vi "CreateVIPictures.vi"(8 "error in (no error)":errorcluster, 9 "Capture Target":T3=enum."Front Panel", 10 "VI Screenshots":T1, 11 "Picture Save Location":path) -> (0 "error out":errorcluster, 2 "Screenshot Files":path[](array[path]))   [LabVIEW 2017]
doc: "Captures .png imgaes of the VI given the path and the picture configuration."
uses:
  Utilities/FilePaths.ctl
  Screenshot Type.ctl
  ScreenshotInfo.ctl
  VIScreenshots.ctl
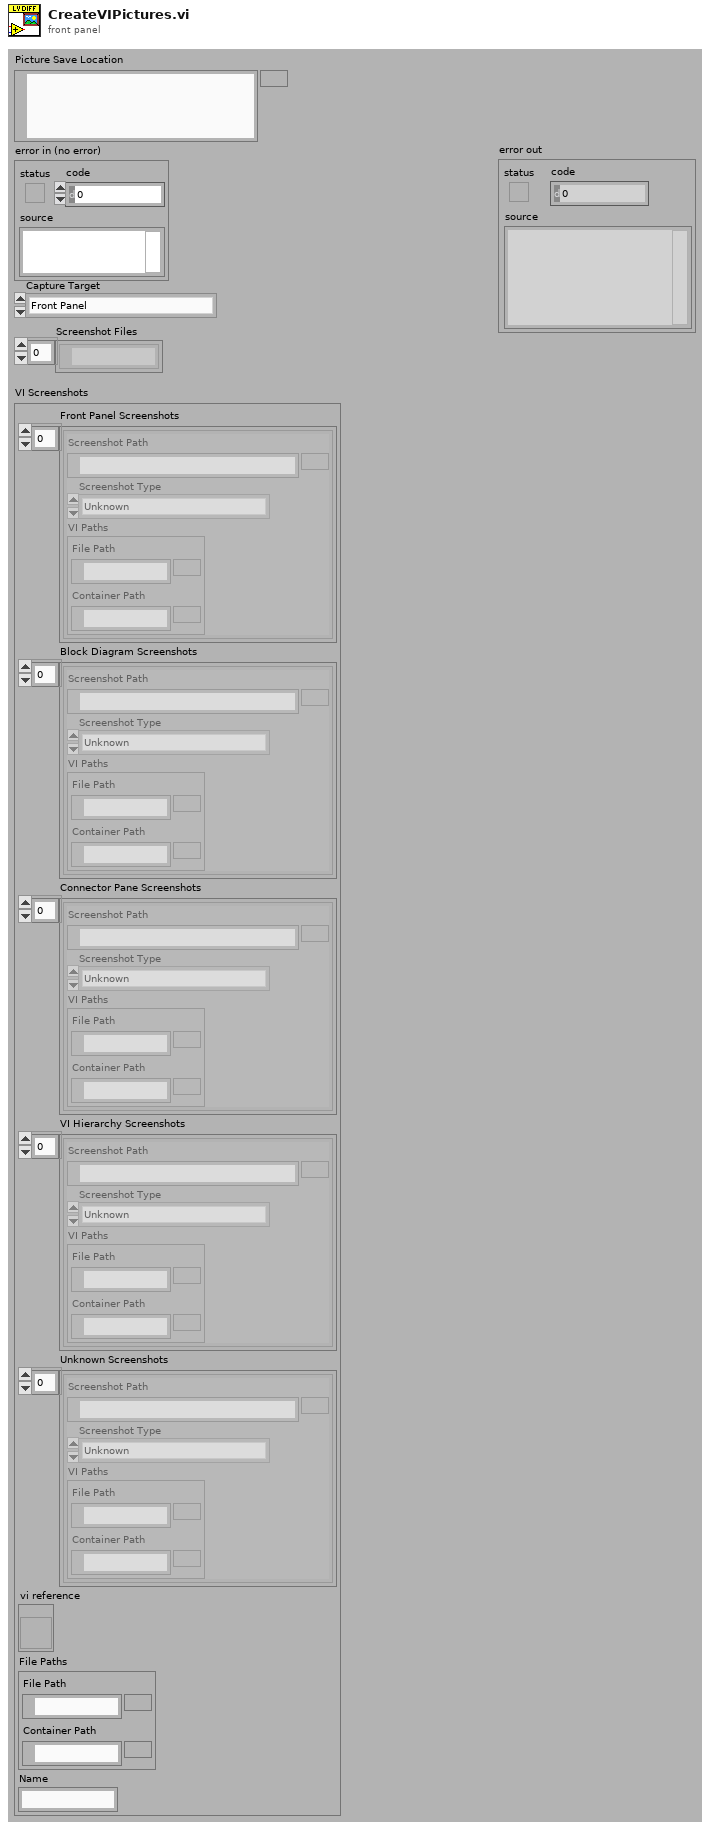
[diagram p1: front panel]
types:
  T1 = typedef "VIScreenshots.ctl" = cluster{"Front Panel Screenshots":T2[], "Block Diagram Screenshots":T2[], "Connector Pane Screenshots":T2[], "VI Hierarchy Screenshots":T2[], "Unknown Screenshots":T2[], "vi reference":refnum<vi>, "File Paths":cluster{"File Path":path, "Container Path":path}, "Name":string}
  T2 = typedef "ScreenshotInfo.ctl" = cluster{"Screenshot Path":path, "Screenshot Type":T3, "VI Paths":T4}
  T3 = typedef "Screenshot Type.ctl" = enum16{"Unknown", "Front Panel", "Connector Pane", "Block Diagram", "VI Hierarchy"}
  T4 = typedef "FilePaths.ctl" = cluster{"File Path":path, "Container Path":path}
  T5 = cluster{"Printing:Custom All Controls?":bool, "Printing:Custom Connector?":bool, "Printing:Custom Control Descriptions?":bool, "Printing:Custom Control Types?":bool, "Printing:Custom Controls?":bool, "Printing:Custom Description?":bool, "Printing:Custom Diagram Hidden?":bool, "Printing:Custom Diagram Repeat?":bool, "Printing:Custom Diagram?":bool, "Printing:Custom Hierarchy?":bool, "Printing:Custom History?":bool, "Printing:Custom Panel Border?":bool, "Printing:Custom Panel?":bool, "Printing:Custom SubVIs?":bool}
  T6 = enum32{"Custom", "Standard", "Using Panel", "Using SubVI", "Complete"}
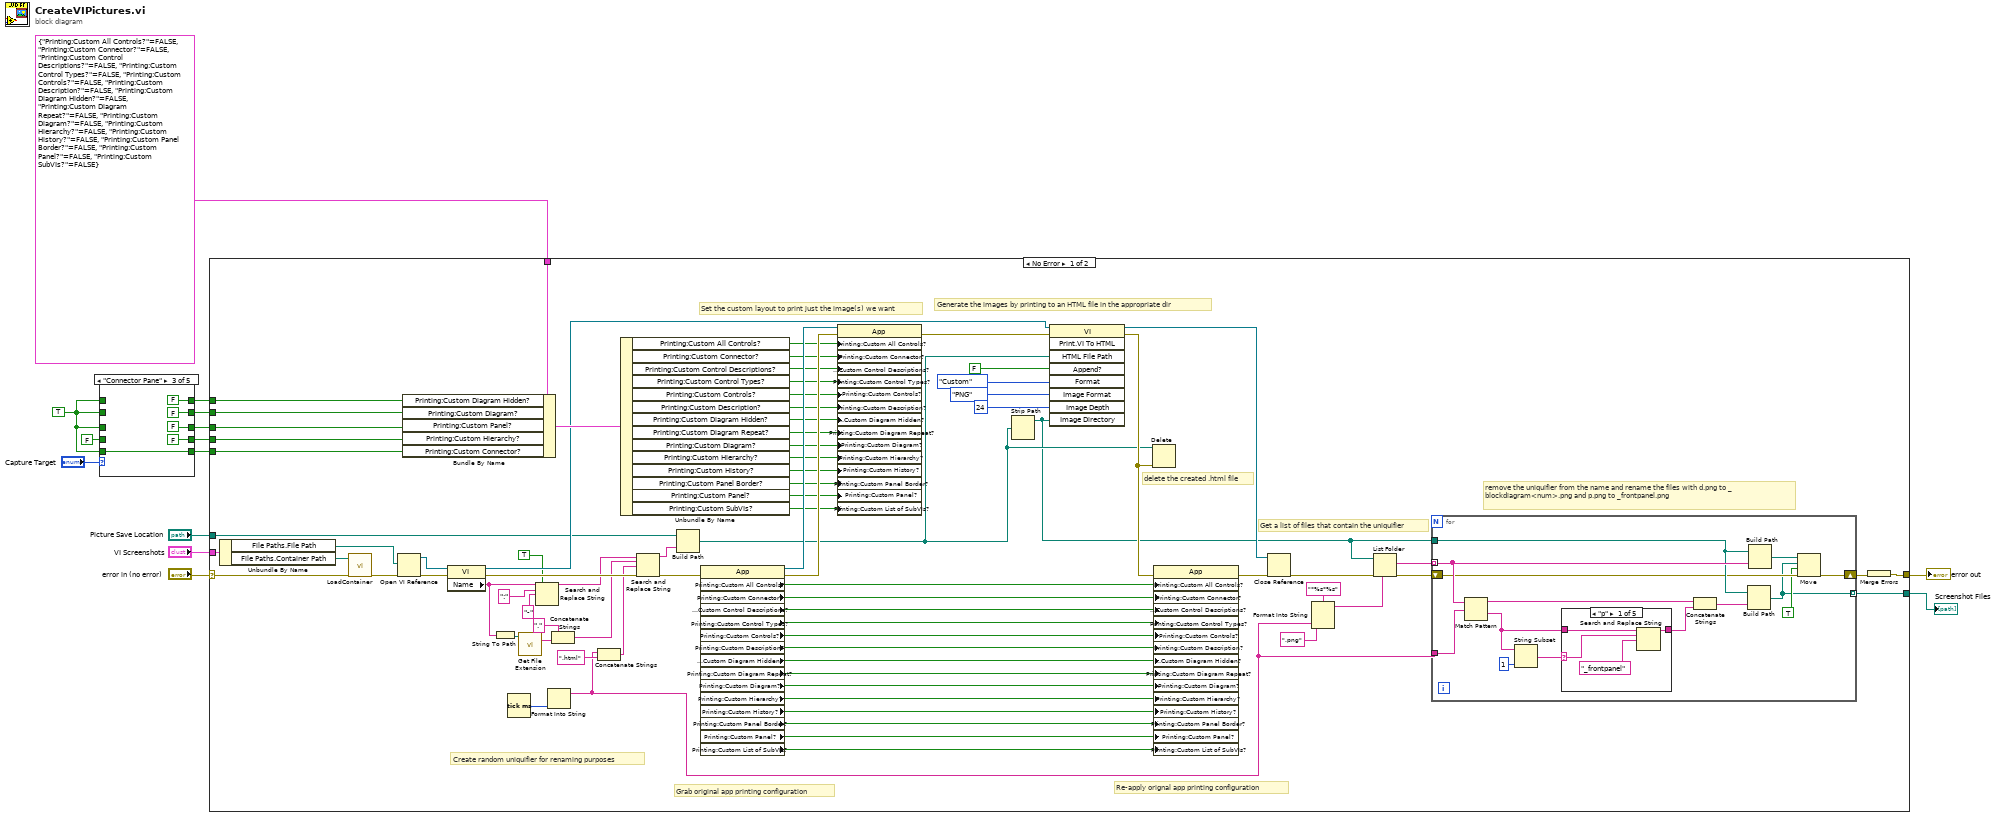
[diagram p0: block diagram]
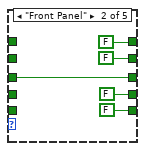
[diagram p3: hidden frame]
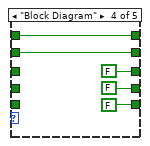
[diagram p4: hidden frame]
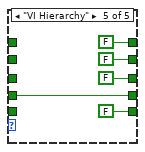
[diagram p5: hidden frame]
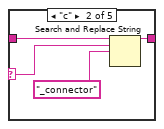
[diagram p6: hidden frame]
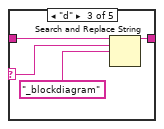
[diagram p7: hidden frame]
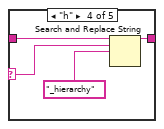
[diagram p8: hidden frame]
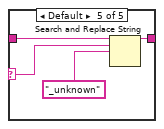
[diagram p9: hidden frame]
diagram:
  w6 = TRUE ("Capture Hierarchy?")
  n1 = case shown="\"Connector Pane\"" "Capture Target" {
    tunnel: FALSE ("Capture Hierarchy?") -> [w19 _ _ _ w35]
    tunnel: w6 -> [w18 _ w28 _ _]
    tunnel: w6 -> [w17 w24 _ _ _]
    tunnel: w6 -> [w16 _ _ w31 _]
    tunnel: w6 -> [w15 _ _ w30 _]
    tunnel: [w19 FALSE ("Capture Hierarchy?") FALSE ("Capture Hierarchy?") FALSE ("Capture Hierarchy?") w35] -> w2
    tunnel: [w18 FALSE ("Capture Connector?") w28 FALSE ("Capture Block Diagram?") FALSE ("Capture Block Diagram?")] -> w1
    tunnel: [w17 w24 FALSE ("Capture Block Diagram?") FALSE ("Capture Block Diagram?") FALSE ("Capture Block Diagram?")] -> w3
    tunnel: [w16 FALSE ("Capture Block Diagram?") FALSE ("Capture Block Diagram?") w31 FALSE ("Capture Block Diagram?")] -> w4
    tunnel: [w15 FALSE ("Capture Hidden Cases?") FALSE ("Capture Hidden Cases?") w30 FALSE ("Capture Block Diagram?")] -> w5
    frame "Unknown", Default {
    }
    frame "Front Panel" {
    }
    frame "Connector Pane" {
    }
    frame "Block Diagram" {
    }
    frame "VI Hierarchy" {
    }
  }
  n2 = case shown="No Error" "error in (no error)" {
    selector: "error in (no error)" -> [w47 w155]
    tunnel: T5 {"Printing:Custom All Controls?"=FALSE, "Printing:Custom Connector?"=FALSE, "Printing:Custom Control Descriptions?"=FALSE, "Printing:Custom Control Types?"=FALSE, "Printing:Custom Controls?"=FALSE, "Printing:Custom Description?"=FALSE, "Printing:Custom Diagram Hidden?"=FALSE, "Printing:Custom Diagram Repeat?"=FALSE, "Printing:Custom Diagram?"=FALSE, "Printing:Custom Hierarchy?"=FALSE, "Printing:Custom History?"=FALSE, "Printing:Custom Panel Border?"=FALSE, "Printing:Custom Panel?"=FALSE, "Printing:Custom SubVIs?"=FALSE} ("Content Options") -> [w120 _]
    tunnel: w5 -> [w119 _]
    tunnel: w4 -> [w118 _]
    tunnel: w3 -> [w117 _]
    tunnel: "Picture Save Location" -> [w78 _]
    tunnel: [w64 w155] -> w12
    tunnel: w2 -> [w63 _]
    tunnel: w1 -> [w62 _]
    tunnel: "VI Screenshots" -> [w49 _]
    tunnel: [w45 _] -> w10
    frame No Error {
      # "remove the uniquifier from the name and rename the files with d.png to _blockdiagram<num>.png and p.png to _frontpanel.png"
      # "Get a list of files that contain the uniquifier"
      # "delete the created .html file"
      # "Create random uniquifier for renaming purposes"
      # "Re-apply orignal app printing configuration"
      # "Grab original app printing configuration"
      # "Generate the images by printing to an HTML file in the appropriate dir"
      # "Set the custom layout to print just the image(s) we want"
      n3 = Unbundle By Name(w49) -> ("File Paths.File Path"=w40:path, "File Paths.Container Path"=w48:path)
      n4 = call "LoadContainer.vi"("error in (no error)"=w47, "Container Path"=w48) -> ("error out"=w43:errorcluster)  [unwired: 9 in]
      n5 = Open VI Reference(vi path=w40, error in (no error)=w43) -> (vi reference=w41:refnum<vi>, error out=w42:errorcluster)  [unwired: 4 in]
      n6 = Bundle By Name(cluster=w120, "Printing:Custom Diagram Hidden?"=w119, "Printing:Custom Diagram?"=w118, "Printing:Custom Panel?"=w117, "Printing:Custom Hierarchy?"=w63, "Printing:Custom Connector?"=w62) -> (w83:T5)
      n7 = property class="VI"(reference=w41, error in=w42) -> (reference out=w79:refnum<vi>, error out=w73:errorcluster, "Name"=w57:string)
      n8 = String To Path(string=w57) -> (path=w61:path)
      n9 = Tick Count (ms)() -> (millisecond timer value=w46:u32)
      n10 = call <vilib>:"Get File Extension.vi"("file"=w61) -> ("lowercase file extension"=w60:string)  [unwired: 6 in, 4 out]
      n11 = Search and Replace String(replace all?=TRUE ("replace all? (F)"), input string=w57, search string=":", replace string="-" ("replace string (\"\")")) -> (result string=w56:string)  [unwired: 4 in, 3 out]
      n12 = Format Into String(w46) -> (resulting string=w53:string)  [unwired: 3 in, 1 out]
      n13 = Concatenate Strings("." ("string"), w60) -> (w58:string)
      n14 = Concatenate Strings(w53, ".html" ("regular expression")) -> (w52:string)
      n15 = Unbundle By Name(w83) -> ("Printing:Custom All Controls?"=w97:bool, "Printing:Custom Connector?"=w96:bool, "Printing:Custom Control Descriptions?"=w95:bool, "Printing:Custom Control Types?"=w94:bool, "Printing:Custom Controls?"=w93:bool, "Printing:Custom Description?"=w92:bool, "Printing:Custom Diagram Hidden?"=w91:bool, "Printing:Custom Diagram Repeat?"=w90:bool, "Printing:Custom Diagram?"=w89:bool, "Printing:Custom Hierarchy?"=w88:bool, "Printing:Custom History?"=w87:bool, "Printing:Custom Panel Border?"=w86:bool, "Printing:Custom Panel?"=w85:bool, "Printing:Custom SubVIs?"=w84:bool)
      n16 = Search and Replace String(input string=w56, search string=w58, replace string=w52, error in=w73) -> (result string=w74:string, error out=w72:errorcluster)  [unwired: 4 in, 2 out]
      n17 = Build Path(base path=w78, name or relative path=w74) -> (appended path=w75:path)
      n18 = property class="App"(error in=w72) -> (reference out=w102:refnum<vi>, error out=w101:errorcluster, "Printing:Custom All Controls?"=w103:bool, "Printing:Custom Connector?"=w104:bool, "Printing:Custom Control Descriptions?"=w105:bool, "Printing:Custom Control Types?"=w106:bool, "Printing:Custom Controls?"=w107:bool, "Printing:Custom Description?"=w108:bool, "Printing:Custom Diagram Hidden?"=w109:bool, "Printing:Custom Diagram Repeat?"=w110:bool, "Printing:Custom Diagram?"=w111:bool, "Printing:Custom Hierarchy?"=w112:bool, "Printing:Custom History?"=w113:bool, "Printing:Custom Panel Border?"=w114:bool, "Printing:Custom Panel?"=w115:bool, "Printing:Custom List of SubVIs?"=w116:bool)  [unwired: 1 in]
      n19 = property class="App"(reference=w102, error in=w101, "Printing:Custom All Controls?"=w97, "Printing:Custom Connector?"=w96, "Printing:Custom Control Descriptions?"=w95, "Printing:Custom Control Types?"=w94, "Printing:Custom Controls?"=w93, "Printing:Custom Description?"=w92, "Printing:Custom Diagram Hidden?"=w91, "Printing:Custom Diagram Repeat?"=w90, "Printing:Custom Diagram?"=w89, "Printing:Custom Hierarchy?"=w88, "Printing:Custom History?"=w87, "Printing:Custom Panel Border?"=w86, "Printing:Custom Panel?"=w85, "Printing:Custom List of SubVIs?"=w84) -> (error out=w100:errorcluster)  [unwired: 1 out]
      n20 = Strip Path(path=w75) -> (stripped path=w67:path)  [unwired: 1 out]
      n21 = invoke class="VI" method="Print.VI To HTML"(reference=w79, error in=w100, "HTML File Path"=w75, "Append?"=FALSE, "Format"=T6."Custom", "Image Format"=enum32{"PNG", "JPEG", "GIF"}."PNG" ("Image Format (jpeg)"), "Image Depth"=24, "Image Directory"=w67) -> (reference out=w76:refnum<vi>, error out=w80:errorcluster)  [unwired: 1 in, 7 out]
      n22 = Delete(path (use dialog)=w75, error in=w80) -> ()  [unwired: 3 in, 3 out]
      n23 = property class="App"(error in=w80, "Printing:Custom All Controls?"=w103, "Printing:Custom Connector?"=w104, "Printing:Custom Control Descriptions?"=w105, "Printing:Custom Control Types?"=w106, "Printing:Custom Controls?"=w107, "Printing:Custom Description?"=w108, "Printing:Custom Diagram Hidden?"=w109, "Printing:Custom Diagram Repeat?"=w110, "Printing:Custom Diagram?"=w111, "Printing:Custom Hierarchy?"=w112, "Printing:Custom History?"=w113, "Printing:Custom Panel Border?"=w114, "Printing:Custom Panel?"=w115, "Printing:Custom List of SubVIs?"=w116) -> (error out=w77:errorcluster)  [unwired: 1 in, 1 out]
      n24 = Close Reference(reference=w76, error in (no error)=w77) -> (error out=w70:errorcluster)
      n25 = Format Into String(format string="*%s*%s" ("Format String"), w53, ".png" ("input 2")) -> (resulting string=w69:string)  [unwired: 2 in, 1 out]
      n26 = List Folder(path=w67, pattern=w69, error in=w70) -> (filenames=w66:string[], error out=w65:errorcluster)  [unwired: 1 in, 2 out]
      n27 = for {
        tunnel: w67 -> [w127]
        tunnel: w66 -> [w128] mode=indexing
        tunnel: w53 -> [w125]
        shift-right: [w123] -> w55
        shift-left: w65 -> [w124]
        tunnel: [w121] -> w45 mode=indexing
        n28 = Match Pattern(string=w128, regular expression=w125) -> (before substring=w130:string, after substring=w132:string)  [unwired: 1 in, 2 out]
        n29 = String Subset(string=w132, length (rest)=1 ("length (rest)")) -> (substring=w133:string)  [unwired: 1 in]
        n30 = case shown="\"p\"" w133 {
          selector: w133 -> [w137 w141 w145 w149 w153]
          tunnel: w132 -> [w138 w142 w146 w150 w154]
          tunnel: [w135 w139 w143 w147 w151] -> w131
          frame "p" {
            n31 = Search and Replace String(input string=w138, search string=w137, replace string="_frontpanel" ("replace string (\"\")")) -> (result string=w135:string)  [unwired: 5 in, 3 out]
          }
          frame "c" {
            n32 = Search and Replace String(input string=w142, search string=w141, replace string="_connector" ("replace string (\"\")")) -> (result string=w139:string)  [unwired: 5 in, 3 out]
          }
          frame "d" {
            n33 = Search and Replace String(input string=w146, search string=w145, replace string="_blockdiagram" ("replace string (\"\")")) -> (result string=w143:string)  [unwired: 5 in, 3 out]
          }
          frame "h" {
            n34 = Search and Replace String(input string=w150, search string=w149, replace string="_hierarchy" ("replace string (\"\")")) -> (result string=w147:string)  [unwired: 5 in, 3 out]
          }
          frame Default {
            n35 = Search and Replace String(input string=w154, search string=w153, replace string="_unknown" ("replace string (\"\")")) -> (result string=w151:string)  [unwired: 5 in, 3 out]
          }
        }
        n36 = Concatenate Strings(w130, w131) -> (w129:string)
        n37 = Build Path(base path=w127, name or relative path=w129) -> (appended path=w121:path)
        n38 = Build Path(base path=w127, name or relative path=w128) -> (appended path=w126:path)
        n39 = Move(source path=w126, error in=w124, 9:TRUE ("overwrite (F)"), 10:w121) -> (error out=w123:errorcluster)  [unwired: 1 in, 2 out]
      }
      n40 = Merge Errors(w55) -> (w64:errorcluster)
    }
    frame Error {
    }
  }
  "error out" <- w12
  "Screenshot Files" <- w10
